vi "File_Save SubVi.vi"(8 "Error":errorcluster, 10 "Default Directory":path, 11 "VI Ref":refnum<vi>) -> (0 "Error Out":errorcluster, 3 "VI Ref Out":refnum<vi>)   [LabVIEW 2009]
doc: "Saves a subvi"
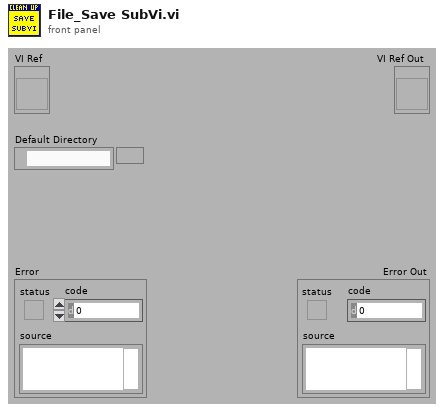
[diagram p1: front panel]
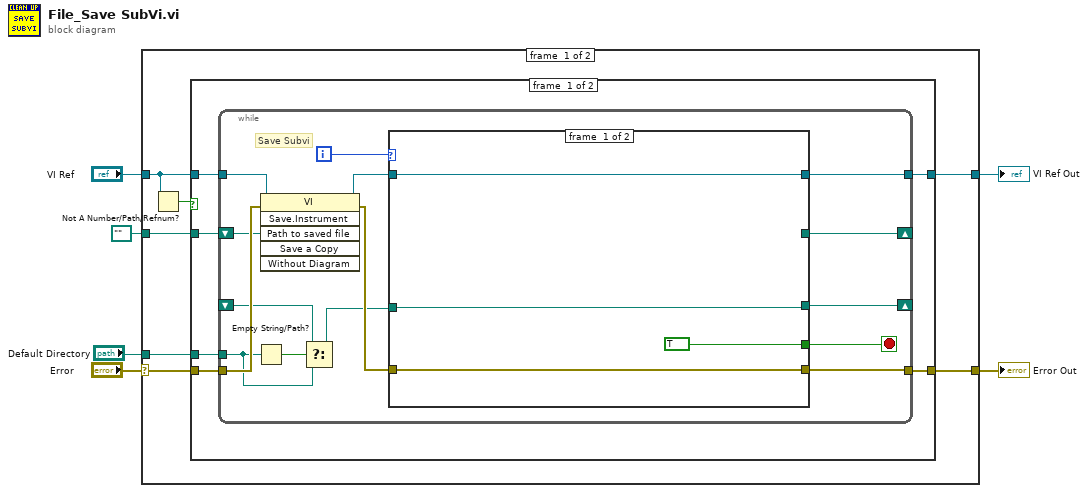
[diagram p0: block diagram]
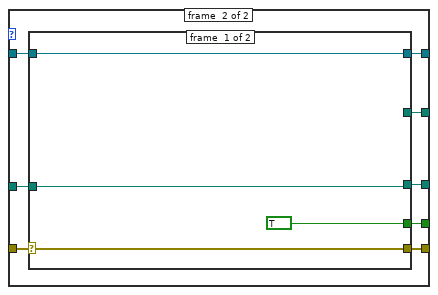
[diagram p2: hidden frame]
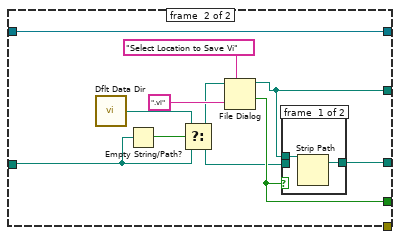
[diagram p3: hidden frame]
diagram:
  n1 = case shown="No Error" "Error" {
    selector: "Error" -> [w10 w67]
    tunnel: [w13 w66] -> w6
    tunnel: [w12 w67] -> w5
    tunnel: "VI Ref" -> [w8 w66]
    tunnel: path "" ("Path to saved file") -> [w11 _]
    tunnel: "Default Directory" -> [w9 _]
    frame #0 {
      n2 = Not A Number/Path/Refnum?(number/path/refnum=w8) -> (NaN/Path/Refnum?=w7:bool)
      n3 = case shown="False" w7 {
        tunnel: [w19 w65] -> w13
        tunnel: [w18 w64] -> w12
        tunnel: w8 -> [w17 w65]
        tunnel: w11 -> [w16 _]
        tunnel: w10 -> [w15 w64]
        tunnel: w9 -> [w14 _]
        frame #0 {
          n4 = while {
            tunnel: [w30] -> w19
            tunnel: [w32] -> w18
            tunnel: w17 -> [w29]
            tunnel: w15 -> [w34]
            shift-right: [w21] -> _
            shift-left: w16 -> [w27]
            shift-right: [w20] -> _
            shift-left: _ -> [w22]
            tunnel: w14 -> [w24]
            i -> [w31]
            stop <- w26 stop-if-true
            # "Save Subvi"
            n5 = Empty String/Path?(string/path=w24) -> (empty?=w25:bool)
            n6 = invoke class="VI" method="Save.Instrument"(reference=w29, error in=w34, "Path to saved file"=w27) -> (reference out=w28:refnum<vi>, error out=w33:errorcluster)  [unwired: 3 in, 4 out]
            n7 = Select(t=w22, s=w25, f=w24) -> (s? t:f=w23:path)
            n8 = case shown="0" w31 {
              tunnel: w33 -> [w37 w46]
              tunnel: [w37 w45] -> w32
              tunnel: w28 -> [w38 w44]
              tunnel: [w38 w43] -> w30
              tunnel: [TRUE w42] -> w26
              tunnel: [_ w41] -> w21
              tunnel: w23 -> [w35 w40]
              tunnel: [w35 w39] -> w20
              frame #0 {
              }
              frame #1 {
                n9 = case shown="Error" w46 {
                  selector: w46 -> [w49 _]
                  tunnel: [w49 _] -> w45
                  tunnel: w44 -> [w50 w60]
                  tunnel: [w50 w60] -> w43
                  tunnel: [TRUE w55] -> w42
                  tunnel: [_ w54] -> w41
                  tunnel: w40 -> [w47 w52]
                  tunnel: [w47 w53] -> w39
                  frame #0 {
                  }
                  frame #1 {
                    n10 = call <vilib>:"Dflt Data Dir.vi"() -> ("App:Default Data Directory"=w57:path)
                    n11 = Empty String/Path?(string/path=w52) -> (empty?=w56:bool)
                    n12 = Select(t=w57, s=w56, f=w52) -> (s? t:f=w51:path)
                    n13 = File Dialog(6:".vi" ("pattern"), 7:"Select Location to Save Vi" ("prompt"), 11:w51) -> (1:w55:bool, 3:w54:path)  [unwired: 4 in, 2 out]
                    n14 = case shown="False" w55 {
                      tunnel: w54 -> [w62 _]
                      tunnel: [w61 w63] -> w53
                      tunnel: w51 -> [_ w63]
                      frame #0 {
                        n15 = Strip Path(path=w62) -> (stripped path=w61:path)  [unwired: 1 out]
                      }
                      frame #1 {
                      }
                    }
                  }
                }
              }
            }
          }
        }
        frame #1 {
        }
      }
    }
    frame #1 {
    }
  }
  "VI Ref Out" <- w6
  "Error Out" <- w5
